vi "AuMT8852B EUT User-friendly Name.vi"(8 "error in (no error)":errorcluster, 11 "VISA session":refnum<visa-resource-name>) -> (0 "error out":errorcluster, 2 "error code":i32, 3 "VISA session out":refnum<visa-resource-name>, 4 "User-friendly name out":string)   [LabVIEW 2017]
doc: "Anritsu MT8852B Bluetooth Tester\n\nReports the user-friendly name stored in the EUT.\n\nOUTPUTS\nUser-friendly name out - the name reported by the equipment under test."
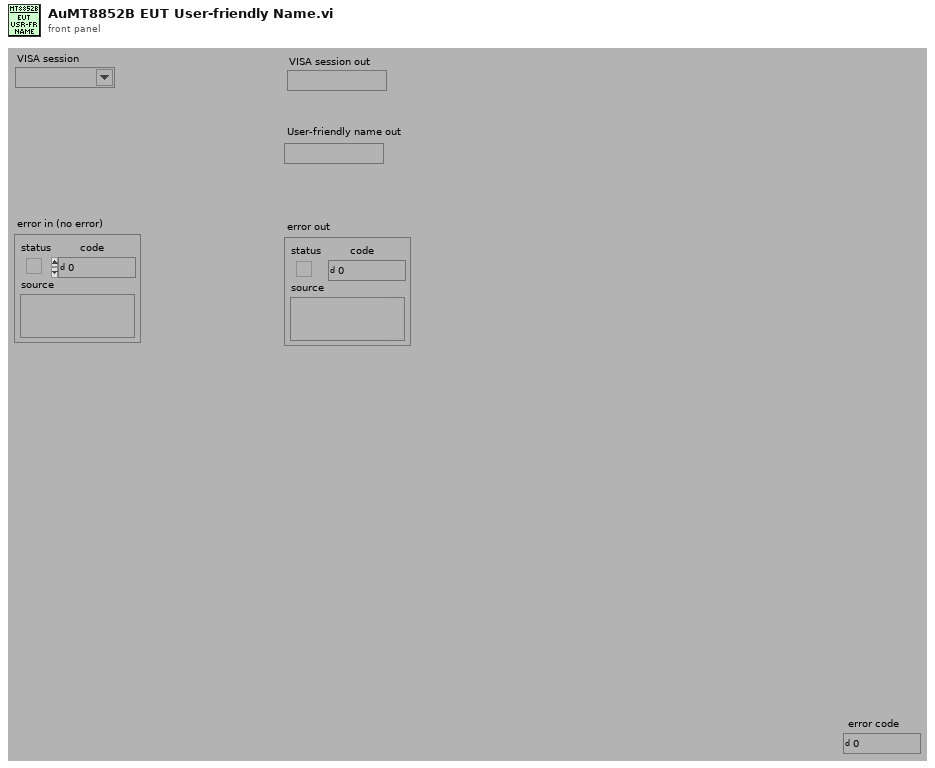
[diagram p1: front panel]
types:
  T1 = enum16{"Simulate", "Range check", "Cache", "Query instrument status"}
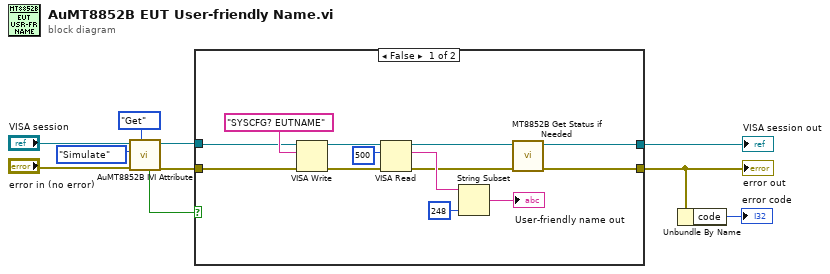
[diagram p0: block diagram]
diagram:
  n1 = call <instrlib>:"AuMT8852B IVI Attribute.vi"("Set/Get (Set)"=enum16{"Set", "Get"}."Get", "error in (no error)"="error in (no error)", "Flag (Simulate)"=T1."Simulate", "VISA session"="VISA session") -> ("error out"=w3:errorcluster, "VISA session out"=w4:refnum<visa-resource-name>, "Value out"=w5:bool)  [unwired: 5 in]
  n2 = case shown="False" w5 {
    tunnel: [w22 w24] -> w1
    tunnel: [w23 w25] -> w10
    tunnel: w4 -> [w13 w25]
    tunnel: w3 -> [w12 w24]
    frame False {
      n3 = VISA Write(VISA resource name=w13, write buffer="SYSCFG? EUTNAME" ("write buffer (\"\")"), error in (no error)=w12) -> (VISA resource name out=w21:refnum<visa-resource-name>, error out=w18:errorcluster)  [unwired: 1 out]
      n4 = VISA Read(VISA resource name=w21, byte count=u32 500 ("byte count (0)"), error in (no error)=w18) -> (VISA resource name out=w15:refnum<visa-resource-name>, read buffer=w17:string, error out=w16:errorcluster)  [unwired: 1 out]
      n5 = String Subset(string=w17, length (rest)=248 ("start index (0)")) -> (substring=→"User-friendly name out":string)  [unwired: 1 in]
      n6 = call <instrlib>:"MT8852B Get Status if Needed.vi"("error in (no error)"=w16, "VISA session"=w15) -> ("error out"=w22:errorcluster, "VISA session out"=w23:refnum<visa-resource-name>)  [unwired: 8 in]
    }
    frame True {
    }
  }
  "error out" <- w1
  "VISA session out" <- w10
  n7 = Unbundle By Name(w1) -> ("code"=→"error code":i32)
